vi "String as UTF-8 String.vi"   [LabVIEW 2020, in "G-Unicode.lvlib"]
doc: "Converts the input string to a UTF-8 encoded LabVIEW string. Valid inputs are a UTF-8 String class or LabVIEW string."
uses:
  G-Unicode.lvlib
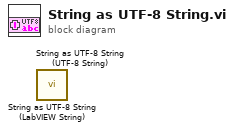
[diagram p0: block diagram]
diagram:
  n1 = call "String as UTF-8 String (LabVIEW String).vi"() -> ()  [unwired: 10 in, 2 out]
  n2 = call "String as UTF-8 String (UTF-8 String).vi"() -> ()  [unwired: 10 in, 2 out]
